vi "HeaterRead.vi"(8 "Error In":errorcluster, 11 "Omega CSi32 In":refnum<visa-resource-name>) -> (0 "Error Out":errorcluster, 2 "Temperature (C)":dbl, 3 "Omega CSi32 Out":refnum<visa-resource-name>)   [LabVIEW 2012]
uses:
  libs/Omega-CSi32/Omega-CSi32.lvlib
  libs/LV-Utilities/LV-Utilities.lvlib
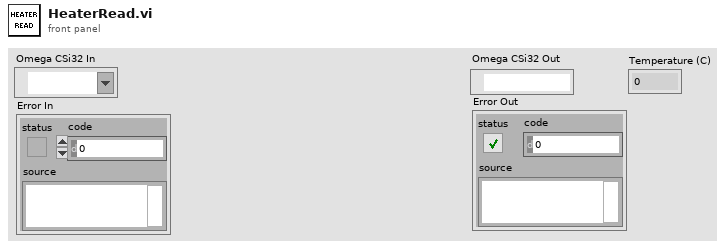
[diagram p1: front panel]
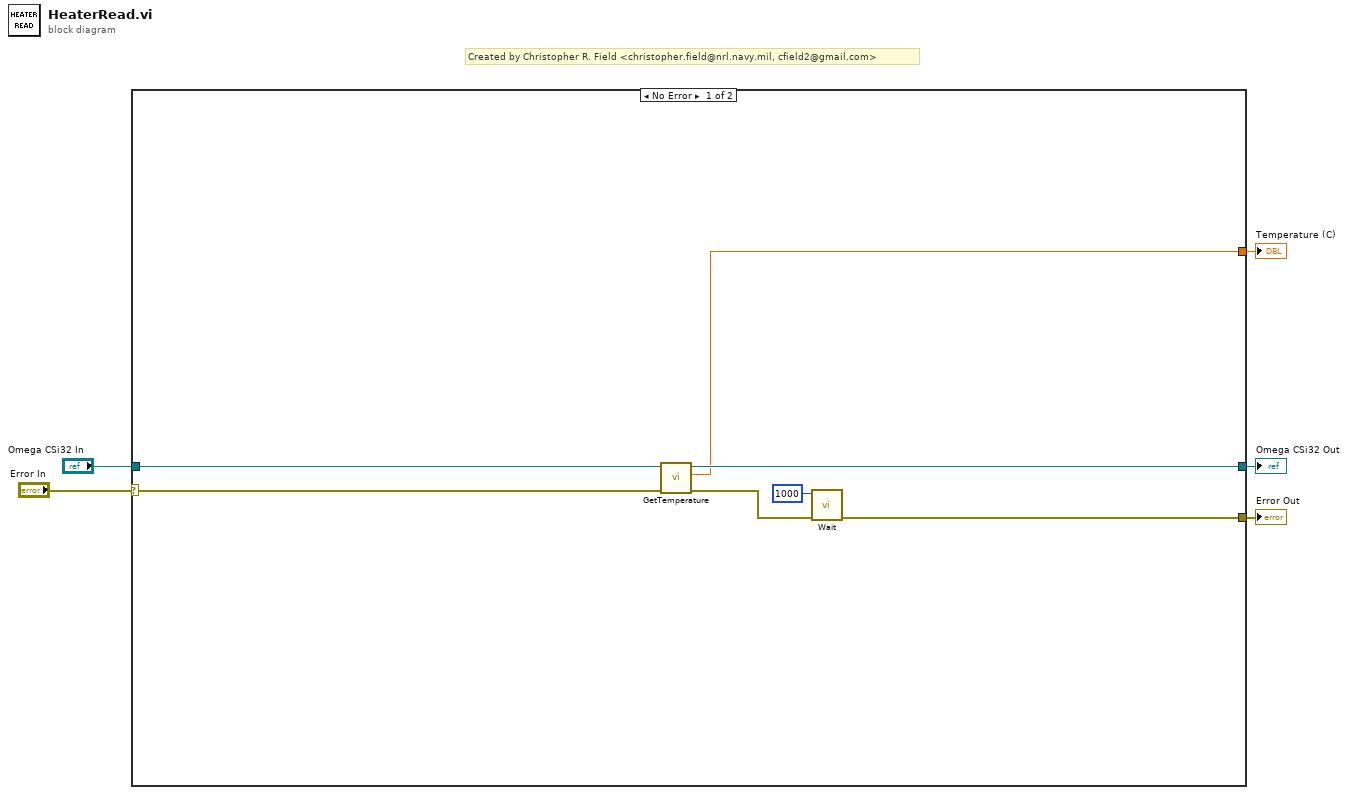
[diagram p0: block diagram]
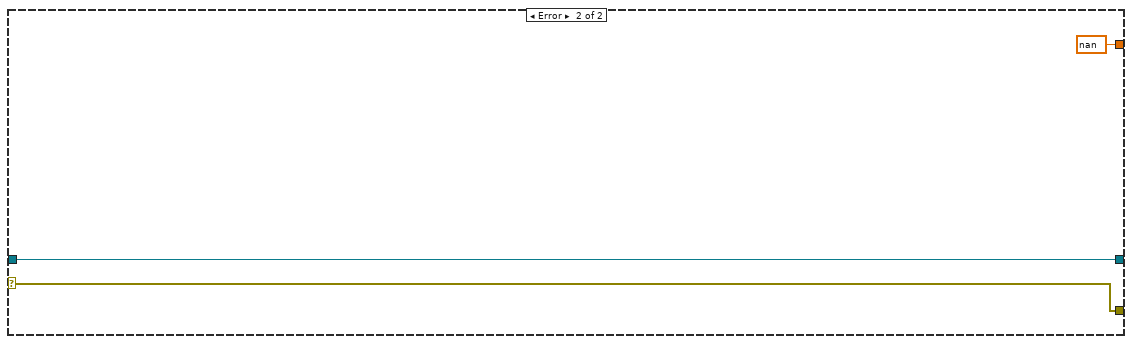
[diagram p2: hidden frame]
diagram:
  # "Created by Christopher R. Field <christopher.field@nrl.navy.mil, cfield2@gmail.com>"
  n1 = case shown="No Error" "Error In" {
    selector: "Error In" -> [w9 w14]
    tunnel: "Omega CSi32 In" -> [w10 w15]
    tunnel: [w8 w15] -> w3
    tunnel: [w7 w14] -> w2
    tunnel: [w6 nan ("Temperature (C)")] -> w1
    frame No Error {
      n2 = call "GetTemperature.vi"("Error In"=w9, "Omega CSi32 In"=w10) -> ("Error Out"=w12:errorcluster, "Temperature (C)"=w6:dbl, "Omega CSi32 Out"=w8:refnum<visa-resource-name>)  [unwired: 6 in, 1 out]
      n3 = call "Wait.vi"("Error In"=w12, "Wait Time (msec)"=u32 1000) -> ("Error Out"=w7:errorcluster)  [unwired: 9 in]
    }
    frame Error {
    }
  }
  "Omega CSi32 Out" <- w3
  "Error Out" <- w2
  "Temperature (C)" <- w1
